vi "CalcDiscrepancy.vi"() -> (0 "output file":path=path "/home/atlas/Micromegas/ProdData/C_CCD/CalcDiscr.txt", 1 "Read Mask File":string="Results*.txt", 2 "Calbration File":string="calib_table.txt")   [LabVIEW 2015]
uses:
  <vilib>/Utility/file.llb/Read Delimited Spreadsheet (string).vi
  GlobalData.vi
  <vilib>/Utility/file.llb/Write Delimited Spreadsheet (DBL).vi
panel:
  out "Path":path
  in  "Table (T)/ stiffback(F)":bool
  in  "stop":bool
  out "ylos 4":dbl
  out "ylos 6":dbl
  out "n":dbl[](array[numeric])
  out "ym":dbl[](array[numeric])
  out "xm":dbl[](array[numeric])
  out "yc":dbl[](array[numeric])
  out "x c":dbl[](array[numeric])
  out "?":dbl
  out "appended array":dbl[][](array[numeric])
  out "y":dbl[](array[numeric])
  out "x":dbl[](array[numeric])
  out "y":dbl
  out "x":dbl
  out "element 3":dbl
  out "element 2":dbl
  out "Misura pannello":string[][](table)
  out "Calibrazione":string[][](table)
  out "element 1":dbl
  out "element":dbl
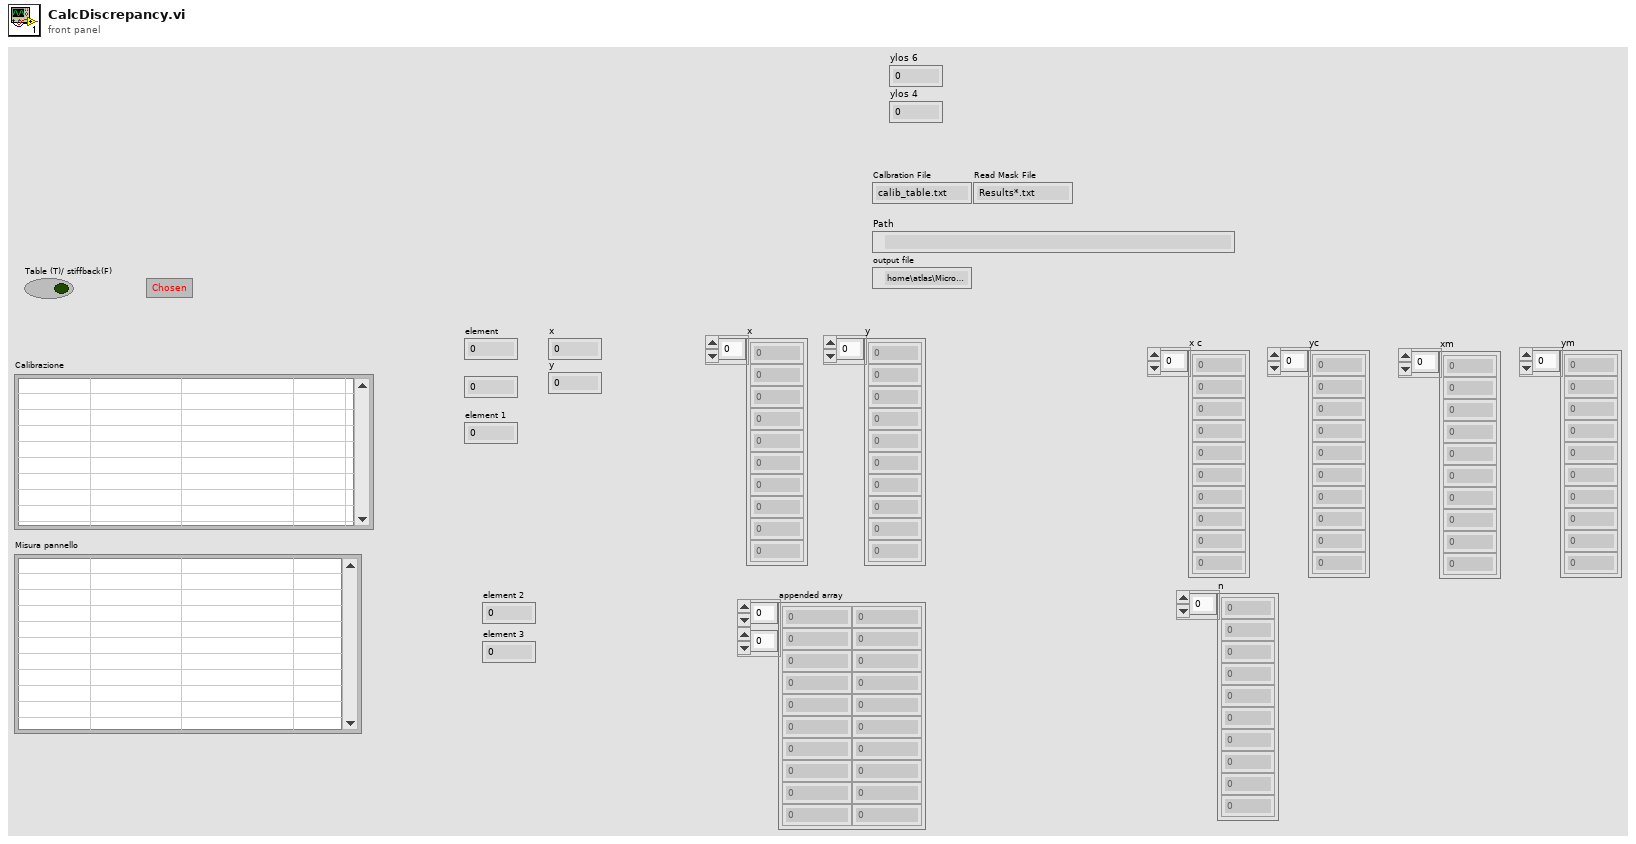
[diagram p1: front panel]
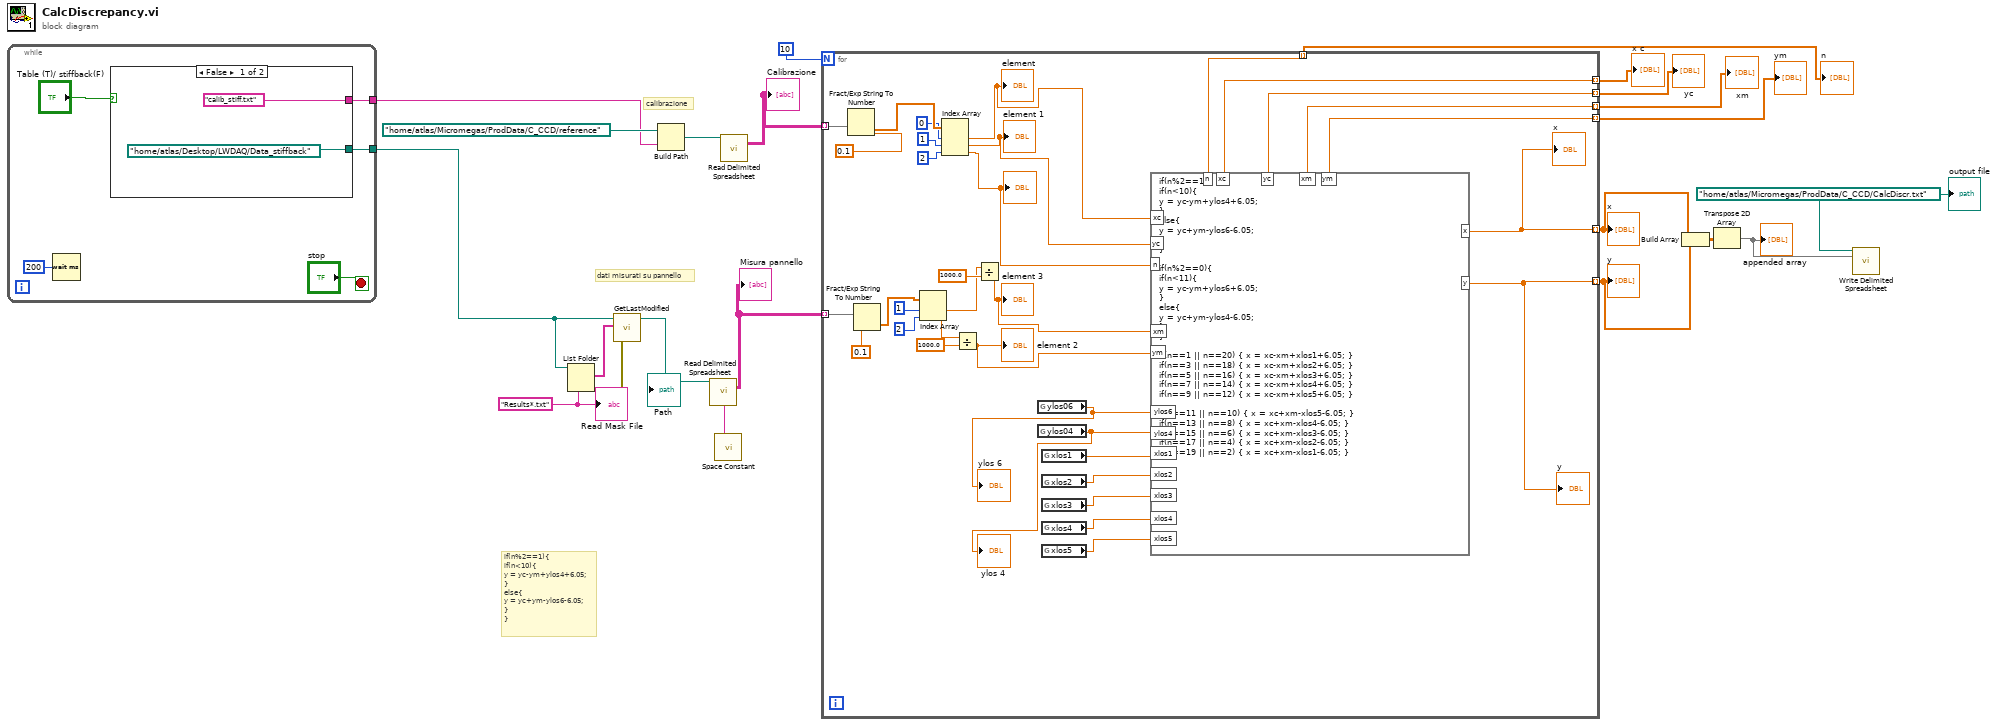
[diagram p0: block diagram]
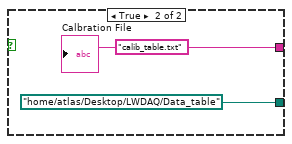
[diagram p2: hidden frame]
diagram:
  w8 = "Results*.txt"
  w11 = path "/home/atlas/Micromegas/ProdData/C_CCD/CalcDiscr.txt" ("file path (dialog if empty)")
  # "if(n%2==1){\nif(n<10){\ny = yc-ym+ylos4+6.05;\n}\nelse{\ny = yc+ym-ylos6-6.05;\n}\n}"
  # "calibrazione"
  # "dati misurati su pannello"
  n1 = while {
    tunnel: [w24] -> w7
    tunnel: [w23] -> w6
    stop <- "stop" stop-if-true
    n2 = Wait (ms)(milliseconds to wait=u32 200) -> ()  [unwired: 1 out]
    n3 = case shown="False" "Table (T)/ stiffback(F)" {
      tunnel: ["calib_stiff.txt" w31] -> w24
      tunnel: [path "/home/atlas/Desktop/LWDAQ/Data_stiffback" ("file path (dialog if empty)") path "/home/atlas/Desktop/LWDAQ/Data_table" ("file path (dialog if empty)")] -> w23
      frame False {
      }
      frame True {
        w31 = "calib_table.txt"
        "Calbration File" <- w31
      }
    }
  }
  n4 = List Folder(path=w6, pattern=w8) -> (filenames=w10:string[], error out=w9:errorcluster)  [unwired: 2 in, 2 out]
  n5 = call "GetLastModified.vi"("error in"=w9, "filenames"=w10, "SearchDir"=w6) -> ("Path"=w5:path)  [unwired: 2 out]
  "Path" <- w5
  n6 = Build Path(base path=path "/home/atlas/Micromegas/ProdData/C_CCD/reference" ("file path (dialog if empty)"), name or relative path=w7) -> (appended path=w2:path)
  n7 = call <vilib>:"Space Constant.vi"() -> ("String"=w3:string)
  n8 = call-poly <vilib>:"Read Delimited Spreadsheet.vi"("file path (dialog if empty)"=w5, "delimiter (\\t)"=w3) -> ("all rows"=w4:string[][])  [unwired: 8 in, 5 out]
  "Misura pannello" <- w4
  n9 = call-poly <vilib>:"Read Delimited Spreadsheet.vi"("file path (dialog if empty)"=w2) -> ("all rows"=w1:string[][])  [unwired: 9 in, 5 out]
  "Calibrazione" <- w1
  n10 = for {
    N: 10 -> [_]
    tunnel: w1 -> [w65] mode=indexing
    tunnel: w4 -> [w62] mode=indexing
    tunnel: [w61] -> w21 mode=indexing
    tunnel: [w60] -> w20 mode=indexing
    tunnel: [w49] -> w16 mode=indexing
    tunnel: [w48] -> w15 mode=indexing
    tunnel: [w46] -> w14 mode=indexing
    tunnel: [w45] -> w13 mode=indexing
    tunnel: [w47] -> w12 mode=indexing
    n11 = Fract/Exp String To Number(string=w65, default (0 dbl)=0.1 ("default (0 DBL)")) -> (number=w59:dbl[])  [unwired: 2 in, 1 out]
    n12 = Fract/Exp String To Number(string=w62, default (0 dbl)=0.1 ("default (0 DBL)")) -> (number=w50:dbl[])  [unwired: 2 in, 1 out]
    n13 = Index Array(array=w50, index #1=1, index #2=2) -> (element #1=w32:dbl, element #2=w36:dbl)
    n14 = Index Array(array=w59, index #1=0, index #2=1, index #3=2) -> (element #1=w55:dbl, element #2=w54:dbl, element #3=w53:dbl)
    "element" <- w55
    "element 1" <- w54
    "?" <- w53
    n15 = Divide(x=w36, y=1000.0) -> (x/y=w37:dbl)
    "element 2" <- w37
    n16 = Divide(x=w32, y=1000.0) -> (x/y=w33:dbl)
    "element 3" <- w33
    n17 = global read "GlobalData.vi" "ylos06"() -> (w39:dbl)
    "ylos 6" <- w39
    n18 = global read "GlobalData.vi" "ylos04"() -> (w38:dbl)
    "ylos 4" <- w38
    n19 = global read "GlobalData.vi" "xlos1"() -> (w44:dbl)
    n20 = global read "GlobalData.vi" "xlos2"() -> (w43:dbl)
    n21 = global read "GlobalData.vi" "xlos3"() -> (w42:dbl)
    n22 = global read "GlobalData.vi" "xlos4"() -> (w41:dbl)
    n23 = global read "GlobalData.vi" "xlos5"() -> (w40:dbl)
    n24 = formula code="if(n%2==1){\nif(n<10){\ny = yc-ym+ylos4+6.05;\n}\nelse{\ny = yc+ym-ylos6-6.05;\n}\n}\n\nif(n%2==0){\nif(n<11){\ny = yc-ym+ylos6+6.05;\n}\nelse{\ny = yc+ym-ylos4-6.05;\n}\n}\n\nif(n==1 || n==20) { x = xc-xm+xlos1+6.05; } \nif(n==3 || n==18) { x = xc-xm+xlos2+6.05; }\nif(n==5 || n==16) { x = xc-xm+xlos3+6.05; }\nif(n==7 || n==14) { x = xc-xm+xlos4+6.05; }\nif(n==9 || n==12) { x = xc-xm+xlos5+6.05; }\n\nif(n==11 || n==10) { x = xc+xm-xlos5-6.05; } \nif(n==13 || n==8) { x = xc+xm-xlos4-6.05; }\nif(n==15 || n==6) { x = xc+xm-xlos3-6.05; }\nif(n==17 || n==4) { x = xc+xm-xlos2-6.05; }\nif(n==19 || n==2) { x = xc+xm-xlos1-6.05; }"("xc"=w55, "xm"=w33, "ym"=w37, "yc"=w54, "n"=w53, "ylos6"=w39, "ylos4"=w38, "xlos1"=w44, "xlos2"=w43, "xlos3"=w42, "xlos4"=w41, "xlos5"=w40) -> ("x"=w61:dbl, "y"=w60:dbl, "xc"=w49:dbl, "yc"=w48:dbl, "xm"=w46:dbl, "ym"=w45:dbl, "n"=w47:dbl)
    "x" <- w61
    "y" <- w60
  }
  "x" <- w21
  "y" <- w20
  "x c" <- w16
  "yc" <- w15
  "xm" <- w14
  "ym" <- w13
  "n" <- w12
  n25 = Build Array(w21, w20) -> (w19:dbl[][])
  n26 = Transpose 2D Array(2D array=w19) -> (transposed array=w18:dbl[][])
  "appended array" <- w18
  n27 = call-poly <vilib>:"Write Delimited Spreadsheet.vi"("file path (dialog if empty)"=w11, "2D data"=w18) -> ()  [unwired: 12 in, 2 out]
  "Read Mask File" <- w8
  "output file" <- w11
